vi "Write Path Section.vi"(7 "LC Type":T1, 8 "error in (no error)":errorcluster, 10 "paths":string[](array[string]), 11 "FP-TC-Shared in":refnum<class "FP-TC-Shared.lvclass">) -> (0 "error out":errorcluster, 3 "FP-TC-Shared out":refnum<class "FP-TC-Shared.lvclass">)   [LabVIEW 2019, in "FP-TC-Shared.lvclass"]
uses:
  FP-TC-Shared.lvclass
  typedefs/LC Type--Enum.ctl
  FP-TC-Shared.lvclass/FP-TC-Shared.ctl
  <vilib>/Utility/config.llb/NI_LVConfig.lvlib
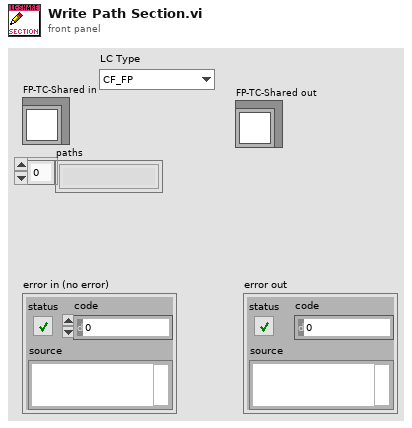
[diagram p1: front panel]
types:
  T1 = typedef "FP-TC-Shared.lvclass/LC Type--Enum.ctl" = enum16{"CF_FP", "CF_TC", "CF_TC_Z", "MNK_FP", "MNK_TC", "MNK_TC_Z"}
  T2 = typedef "NI_LVConfig.lvlib/Config Data RefNum.ctl" = refnum<k1>
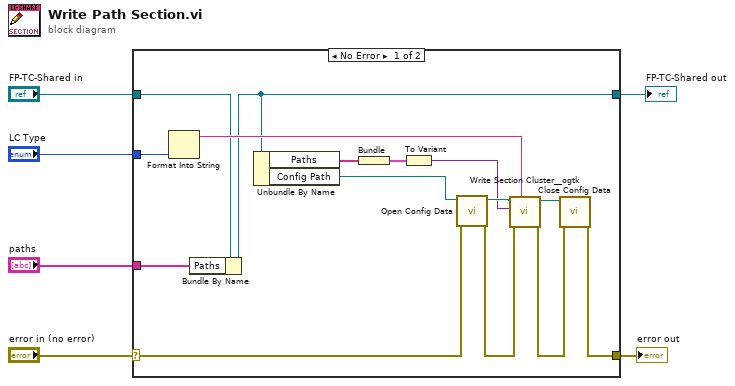
[diagram p0: block diagram]
diagram:
  n1 = case shown="No Error" "error in (no error)" {
    selector: "error in (no error)" -> [w20 w23]
    tunnel: "paths" -> [w10 _]
    tunnel: [w21 w23] -> w5
    tunnel: "FP-TC-Shared in" -> [w8 w22]
    tunnel: "LC Type" -> [w14 _]
    tunnel: [w9 w22] -> w1
    frame No Error {
      n2 = Format Into String(w14) -> (resulting string=w13:string)  [unwired: 3 in, 1 out]
      n3 = Bundle By Name(cluster=w8, "Paths"=w10) -> (w9:refnum<class "FP-TC-Shared.lvclass">)
      n4 = Unbundle By Name(w9) -> ("Paths"=w7:string[], "Config Path"=w19:path)
      n5 = Bundle("Paths"=w7) -> (w12:cluster{"Paths":string[]})  [unwired: 1 in]
      n6 = To Variant(anything=w12) -> (Variant=w11:variant)
      n7 = call <vilib>:"Open Config Data.vi"("error in (no error)"=w20, "configuration file path"=w19) -> ("error out"=w15:errorcluster, "refnum"=w16:T2)  [unwired: 7 in, 1 out]
      n8 = call <userlib>:"Write Section Cluster__ogtk.vi"("section (optional)"=w13, "error in (no error)"=w15, "Section Formatted Cluster"=w11, "refnum"=w16) -> ("error out"=w17:errorcluster, "dup refnum"=w18:T2)  [unwired: 6 in]
      n9 = call <vilib>:"Close Config Data.vi"("error in (no error)"=w17, "refnum"=w18) -> ("error out"=w21:errorcluster)  [unwired: 8 in, 1 out]
    }
    frame Error {
    }
  }
  "error out" <- w5
  "FP-TC-Shared out" <- w1
